vi "Prompt_EventExists.vi"(5 "Project Strings":string[](array[string]), 6 "Measurement number":i32=8, 7 "Meas. Description":string="200C", 8 "SubFolder":string="Temp Dependence", 9 "Project":u16(ring) items=["Unspecified", "Proj_VaporTubes", "Proj_H2DT", "Proj_PIHVOF", "Proj_PIHVOF2"]) -> (1 "Meas. Description 2":string="200C", 2 "SubFolder 2":string="Temp Dependence", 3 "Project 2":u16(ring) items=["H2TC", "VAPOR1"], 4 "Measurement number 2":i32=8)   [LabVIEW 2018]
doc: "Displays a standard dialog box that prompts users to enter information, such as a user name and password.\n--------------------\n\nThis Express VI is configured as follows:\n\nMessage to Display to the User:\nThe inputs are: \nText Entry Box: Project\nText Entry Box: Measurement Description\nNumber: Measurement Number"
panel:
  out "String 2":string="Change information below to generate unique filename or overwrite" caption="String"
  out "error out":errorcluster
  in  "Enable":bool=TRUE
  in  "OK2":bool
  in  "OK1":bool
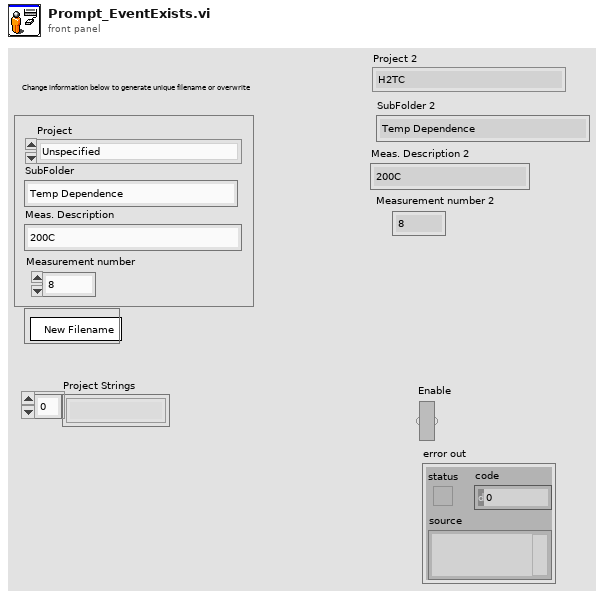
[diagram p1: front panel]
types:
  T1 = cluster{"Input Name":string, "Input Data Type":i32}[]
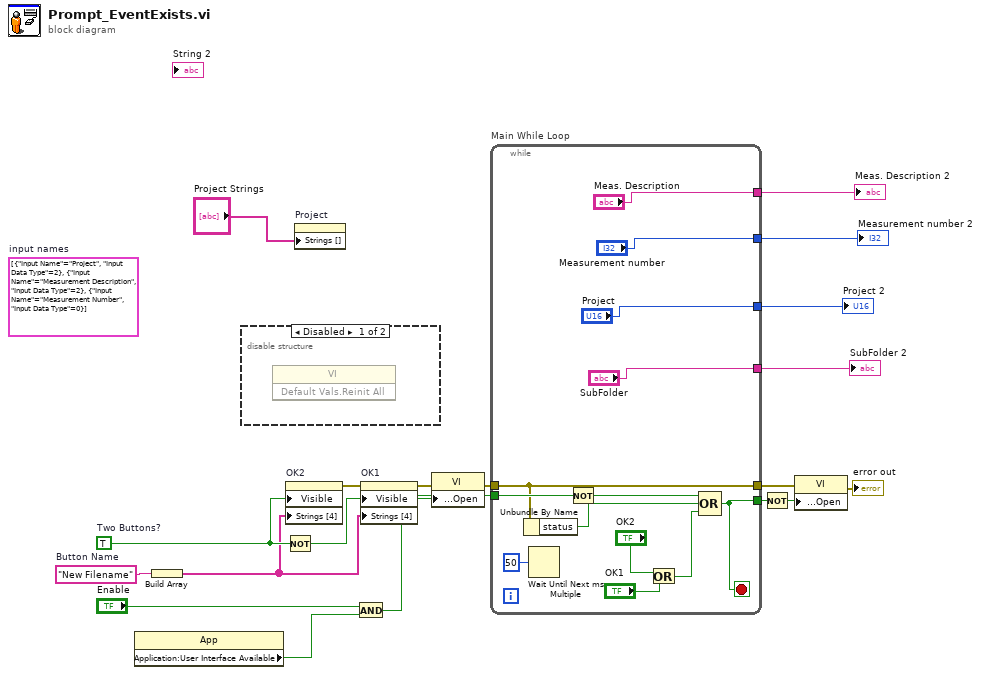
[diagram p0: block diagram]
diagram:
  (unwired) T1 [{"Input Name"="Project", "Input Data Type"=2}, {"Input Name"="Measurement Description", "Input Data Type"=2}, {"Input Name"="Measurement Number", "Input Data Type"=0}]  # input names
  w13 = "New Filename"  # Button Name
  w19 = TRUE  # Two Buttons?
  n1 = property class="App"() -> ("Application:User Interface Available"=w6:bool)  [unwired: 2 in, 2 out]
  n2 = Build Array(w13) -> (w14:string[])
  n3 = disable-structure shown="Disabled" {
    frame Disabled {
      n4 = invoke class="VI" method="Default Vals.Reinit All"() -> ()  [unwired: 3 in, 3 out]
    }
    frame Enabled {
    }
  }
  n5 = Not(x=w19) -> (.not. x?=w18:bool)
  n6 = property on="OK2" class="Bool"("Visible"=w19, "Strings [4]"=w14) -> (error out=w17:errorcluster)  [unwired: 2 in, 1 out]
  n7 = property on="Project" class="Ring (strict)"("Strings []"="Project Strings") -> ()  [unwired: 2 in, 2 out]
  n8 = And(x="Enable", y=w6) -> (x .and. y?=w7:bool)
  n9 = property on="OK1" class="Bool"(error in=w17, "Visible"=w18, "Strings [4]"=w14) -> (error out=w12:errorcluster)  [unwired: 1 in, 1 out]
  n10 = property class="VI"(error in=w12, "Front Panel Window:Open"=w7) -> (error out=w11:errorcluster)  [unwired: 1 in, 1 out]
  n11 = while "Main While Loop" {
    tunnel: w7 -> [w28]
    tunnel: [w26] -> w15
    tunnel: w11 -> [w25]
    tunnel: [w25] -> w10
    tunnel: ["Meas. Description"] -> w5
    tunnel: ["Measurement number"] -> w4
    tunnel: ["Project"] -> w3
    tunnel: ["SubFolder"] -> w2
    stop <- w26 stop-if-true
    n12 = Unbundle By Name(w25) -> ("status"=w24:bool)
    n13 = Wait Until Next ms Multiple(millisecond multiple=u32 50) -> ()  [unwired: 1 out]
    n14 = Not(x=w28) -> (.not. x?=w27:bool)
    n15 = Or(x="OK2", y="OK1") -> (x .or. y?=w30:bool)
    n16 = Compound Arithmetic op=OR(w27, w24, w30) -> (w26:bool)
  }
  "Meas. Description 2" <- w5
  "Measurement number 2" <- w4
  "SubFolder 2" <- w2
  "Project 2" <- w3
  n17 = Not(x=w15) -> (.not. x?=w16:bool)
  n18 = property class="VI"(error in=w10, "Front Panel Window:Open"=w16) -> (error out=→"error out":errorcluster)  [unwired: 1 in, 1 out]
